vi "Crop to trigger.vi"(11 "Live":waveform(dbl)) -> (3 "Live data":dbl[](graph))   [LabVIEW 2017, in "DAQ.lvlib"]
uses:
  DAQ.lvlib
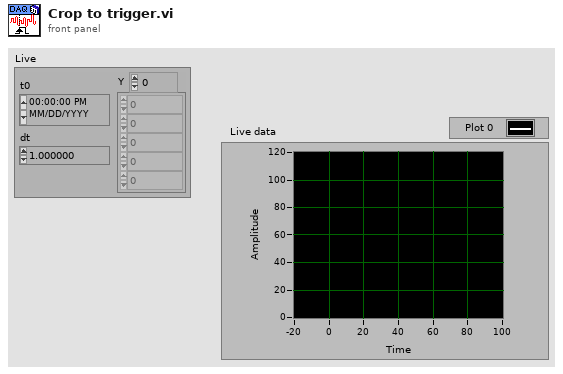
[diagram p1: front panel]
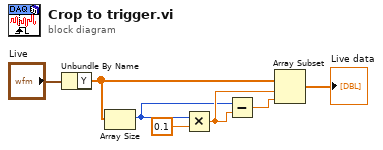
[diagram p0: block diagram]
diagram:
  n1 = Unbundle By Name("Live") -> ("Y"=w7:dbl[])
  n2 = Array Size(array=w7) -> (size(s)=w5:i32)
  n3 = Multiply(x=w5, y=0.1) -> (x*y=w6:dbl)
  n4 = Subtract(x=w5, y=w6) -> (x-y=w4:dbl)
  n5 = Array Subset(array=w7, index=w6, length=w4) -> (→"Live data":dbl[])
